vi "test odczytu TDMS.vi"() -> ()   [LabVIEW 2013]
panel:
  out "group/channel names":string[][](array[string])
  out "group names":string[](array[string])
  in  "file path":path
  out "property names":string[](array[string])
  out "channel name out":string
  out "group name out":string
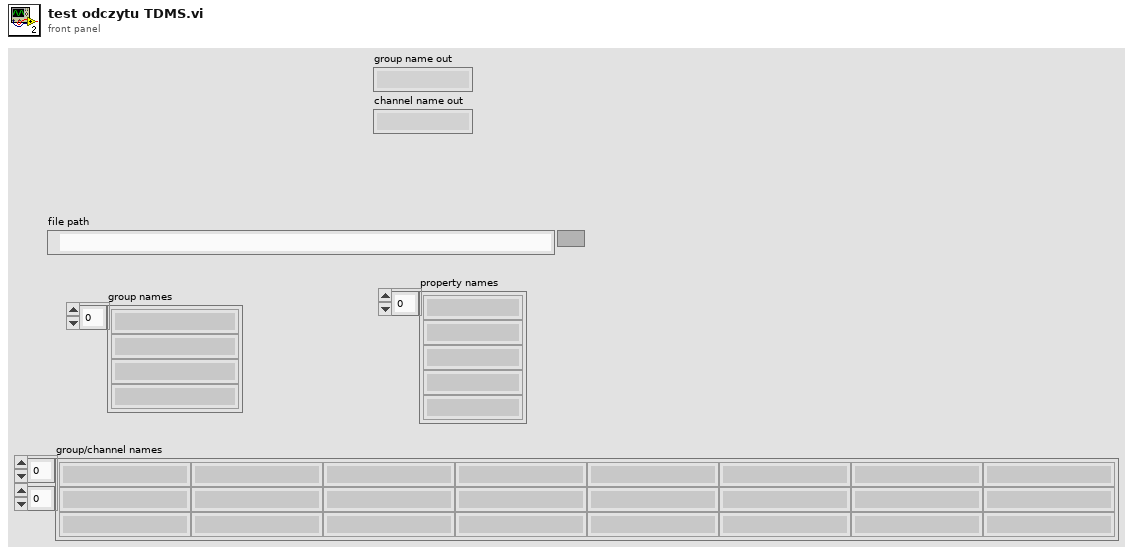
[diagram p1: front panel]
types:
  T1 = enum16{"open", "open or create", "create or replace", "create", "open (read-only)"}
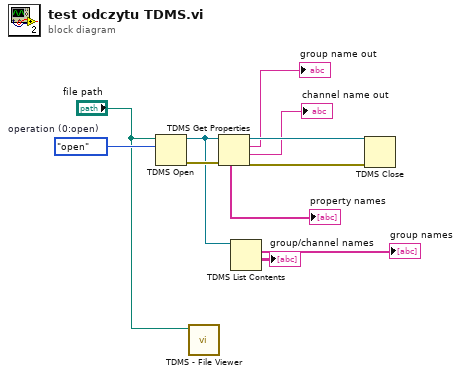
[diagram p0: block diagram]
diagram:
  w10 = T1."open"  # operation (0:open)
  n1 = TDMS Open(10:w10, 11:"file path") -> (0:w11:errorcluster, 3:w4:refnum<k34>)  [unwired: 5 in]
  n2 = call <vilib>:"TDMS - File Viewer.vi"("file path"="file path") -> ()  [unwired: 5 in, 2 out]
  n3 = TDMS Get Properties(8:w11, 11:w4) -> (0:w9:errorcluster, 1:→"channel name out":string, 2:→"group name out":string, 3:w8:refnum<k34>, 6:→"property names":string[])  [unwired: 4 in, 1 out]
  n4 = TDMS List Contents(7:w4) -> (1:→"group/channel names":string[][], 2:→"group names":string[])  [unwired: 2 in, 2 out]
  n5 = TDMS Close(8:w9, 11:w8) -> ()  [unwired: 2 out]
